vi "ELVIS III v1.0 Get Reset Actions.vi"(8 "error in":errorcluster, 11 "String":string) -> (0 "error out":errorcluster, 3 "Resources":string[](array[string]))   [LabVIEW 2021]
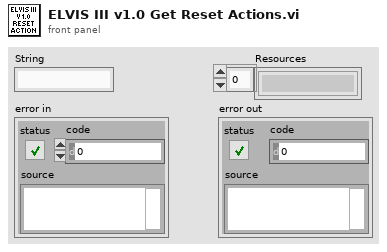
[diagram p1: front panel]
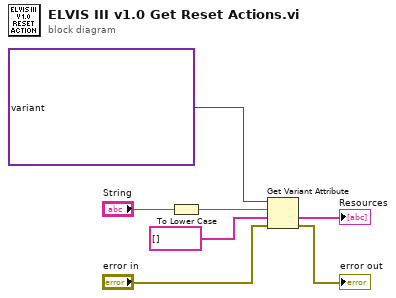
[diagram p0: block diagram]
diagram:
  n1 = To Lower Case(string="String") -> (all lower case string=w6:string)
  n2 = Get Variant Attribute(Variant=variant("a/ai0 (continuous)"=variant(string[] ["No"]), "a/ai0 (diff continuous)"=variant(string[] ["No"]), "a/ai0 (diff n samples)"=variant(string[] ["No"]), "a/ai0 (diff)"=variant(string[] ["No"]), "a/ai0 (interrupt)"=variant(string[] ["No"]), "a/ai0 (n samples)"=variant(string[] ["No"]), "a/ai1"=variant(string[] ["No"]), "a/ai1 (continuous)"=variant(string[] ["No"]), "a/ai1 (diff continuous)"=variant(string[] ["No"]), "a/ai1 (diff n samples)"=variant(string[] ["No"]), "a/ai1 (diff)"=variant(string[] ["No"]), "a/ai1 (interrupt)"=variant(string[] ["No"]), "a/ai1 (n samples)"=variant(string[] ["No"]), "a/ai2"=variant(string[] ["No"]), "a/ai2 (continuous)"=variant(string[] ["No"]), "a/ai2 (diff continuous)"=variant(string[] ["No"]), "a/ai2 (diff n samples)"=variant(string[] ["No"]), "a/ai2 (diff)"=variant(string[] ["No"]), "a/ai2 (n samples)"=variant(string[] ["No"]), "a/ai3"=variant(string[] ["No"]), "a/ai3 (continuous)"=variant(string[] ["No"]), "a/ai3 (diff continuous)"=variant(string[] ["No"]), "a/ai3 (diff n samples)"=variant(string[] ["No"]), "a/ai3 (diff)"=variant(string[] ["No"]), "a/ai3 (n samples)"=variant(string[] ["No"]), "a/ai4"=variant(string[] ["No"]), "a/ai4 (continuous)"=variant(string[] ["No"]), "a/ai4 (n samples)"=variant(string[] ["No"]), "a/ai5"=variant(string[] ["No"]), "a/ai5 (continuous)"=variant(string[] ["No"]), "a/ai5 (n samples)"=variant(string[] ["No"]), "a/ai6"=variant(string[] ["No"]), "a/ai6 (continuous)"=variant(string[] ["No"]), "a/ai6 (n samples)"=variant(string[] ["No"]), "a/ai7"=variant(string[] ["No"]), "a/ai7 (continuous)"=variant(string[] ["No"]), "a/ai7 (n samples)"=variant(string[] ["No"]), "a/ao0"=variant(string[] ["AO"]), "a/ao0 (continuous)"=variant(string[] ["AO DMA", "AO"]), "a/ao0 (n samples)"=variant(string[] ["AO"]), "a/ao1"=variant(string[] ["AO"]), "a/ao1 (continuous)"=variant(string[] ["AO DMA", "AO"]), "a/ao1 (n samples)"=variant(string[] ["AO"]), "a/di0 (n samples)"=variant(string[] ["DI N Samples"]), "a/di1 (n samples)"=variant(string[] ["DI N Samples"]), "a/di10 (n samples)"=variant(string[] ["DI N Samples"]), "a/di11 (n samples)"=variant(string[] ["DI N Samples"]), "a/di12 (n samples)"=variant(string[] ["DI N Samples"]), "a/di13 (n samples)"=variant(string[] ["DI N Samples"]), "a/di14 (n samples)"=variant(string[] ["DI N Samples"]), "a/di15 (n samples)"=variant(string[] ["DI N Samples"]), "a/di16 (n samples)"=variant(string[] ["DI N Samples"]), "a/di17 (n samples)"=variant(string[] ["DI N Samples"]), "a/di18 (n samples)"=variant(string[] ["DI N Samples"]), "a/di19 (n samples)"=variant(string[] ["DI N Samples"]), "a/di2 (n samples)"=variant(string[] ["DI N Samples"]), "a/di3 (n samples)"=variant(string[] ["DI N Samples"]), "a/di4 (n samples)"=variant(string[] ["DI N Samples"]), "a/di5 (n samples)"=variant(string[] ["DI N Samples"]), "a/di6 (n samples)"=variant(string[] ["DI N Samples"]), "a/di7 (n samples)"=variant(string[] ["DI N Samples"]), "a/di8 (n samples)"=variant(string[] ["DI N Samples"]), "a/di9 (n samples)"=variant(string[] ["DI N Samples"]), "a/dio0"=variant(string[] ["DIO"]), "a/dio0 (interrupt)"=variant(string[] ["No"]), "a/dio1"=variant(string[] ["DIO"]), "a/dio1 (interrupt)"=variant(string[] ["No"]), "a/dio10"=variant(string[] ["DIO"]), "a/dio11"=variant(string[] ["DIO"]), "a/dio12"=variant(string[] ["DIO"]), "a/dio13"=variant(string[] ["DIO"]), "a/dio14"=variant(string[] ["DIO"]), "a/dio15"=variant(string[] ["DIO"]), "a/dio16"=variant(string[] ["DIO"]), "a/dio17"=variant(string[] ["DIO"]), "a/dio18"=variant(string[] ["DIO"]), "a/dio19"=variant(string[] ["DIO"]), "a/dio2"=variant(string[] ["DIO"]), "a/dio2 (interrupt)"=variant(string[] ["No"]), "a/dio3"=variant(string[] ["DIO"]), "a/dio3 (interrupt)"=variant(string[] ["No"]), "a/dio4"=variant(string[] ["DIO"]), "a/dio5"=variant(string[] ["DIO"]), "a/dio6"=variant(string[] ["DIO"]), "a/dio7"=variant(string[] ["DIO"]), "a/dio8"=variant(string[] ["DIO"]), "a/dio9"=variant(string[] ["DIO"]), "a/do0 (n samples)"=variant(string[] ["DO N Samples"]), "a/do1 (n samples)"=variant(string[] ["DO N Samples"]), "a/do10 (n samples)"=variant(string[] ["DO N Samples"]), "a/do11 (n samples)"=variant(string[] ["DO N Samples"]), "a/do12 (n samples)"=variant(string[] ["DO N Samples"]), "a/do13 (n samples)"=variant(string[] ["DO N Samples"]), "a/do14 (n samples)"=variant(string[] ["DO N Samples"]), "a/do15 (n samples)"=variant(string[] ["DO N Samples"]), "a/do16 (n samples)"=variant(string[] ["DO N Samples"]), "a/do17 (n samples)"=variant(string[] ["DO N Samples"]), "a/do18 (n samples)"=variant(string[] ["DO N Samples"]), "a/do19 (n samples)"=variant(string[] ["DO N Samples"]), "a/do2 (n samples)"=variant(string[] ["DO N Samples"]), "a/do3 (n samples)"=variant(string[] ["DO N Samples"]), "a/do4 (n samples)"=variant(string[] ["DO N Samples"]), "a/do5 (n samples)"=variant(string[] ["DO N Samples"]), "a/do6 (n samples)"=variant(string[] ["DO N Samples"]), "a/do7 (n samples)"=variant(string[] ["DO N Samples"]), "a/do8 (n samples)"=variant(string[] ["DO N Samples"]), "a/do9 (n samples)"=variant(string[] ["DO N Samples"]), "a/enc0"=variant(string[] ["ENC"]), "a/enc1"=variant(string[] ["ENC"]), "a/enc2"=variant(string[] ["ENC"]), "a/enc3"=variant(string[] ["ENC"]), "a/enc4"=variant(string[] ["ENC"]), "a/enc5"=variant(string[] ["ENC"]), "a/enc6"=variant(string[] ["ENC"]), "a/enc7"=variant(string[] ["ENC"]), "a/enc8"=variant(string[] ["ENC"]), "a/enc9"=variant(string[] ["ENC"]), "a/i2c"=variant(string[] ["I2C"]), "a/pwm0"=variant(string[] ["PWM"]), "a/pwm1"=variant(string[] ["PWM"]), "a/pwm10"=variant(string[] ["PWM"]), "a/pwm11"=variant(string[] ["PWM"]), "a/pwm12"=variant(string[] ["PWM"]), "a/pwm13"=variant(string[] ["PWM"]), "a/pwm14"=variant(string[] ["PWM"]), "a/pwm15"=variant(string[] ["PWM"]), "a/pwm16"=variant(string[] ["PWM"]), "a/pwm17"=variant(string[] ["PWM"]), "a/pwm18"=variant(string[] ["PWM"]), "a/pwm19"=variant(string[] ["PWM"]), "a/pwm2"=variant(string[] ["PWM"]), "a/pwm3"=variant(string[] ["PWM"]), "a/pwm4"=variant(string[] ["PWM"]), "a/pwm5"=variant(string[] ["PWM"]), "a/pwm6"=variant(string[] ["PWM"]), "a/pwm7"=variant(string[] ["PWM"]), "a/pwm8"=variant(string[] ["PWM"]), "a/pwm9"=variant(string[] ["PWM"]), "a/spi"=variant(string[] ["SPI"]), "asrl1::instr"=variant(string[] ["UART"]), "asrl2::instr"=variant(string[] ["UART"]), "b/ai0"=variant(string[] ["No"]), "b/ai0 (continuous)"=variant(string[] ["No"]), "b/ai0 (diff continuous)"=variant(string[] ["No"]), "b/ai0 (diff n samples)"=variant(string[] ["No"]), "b/ai0 (diff)"=variant(string[] ["No"]), "b/ai0 (n samples)"=variant(string[] ["No"]), "b/ai1"=variant(string[] ["No"]), "b/ai1 (continuous)"=variant(string[] ["No"]), "b/ai1 (diff continuous)"=variant(string[] ["No"]), "b/ai1 (diff n samples)"=variant(string[] ["No"]), "b/ai1 (diff)"=variant(string[] ["No"]), "b/ai1 (n samples)"=variant(string[] ["No"]), "b/ai2"=variant(string[] ["No"]), "b/ai2 (continuous)"=variant(string[] ["No"]), "b/ai2 (diff continuous)"=variant(string[] ["No"]), "b/ai2 (diff n samples)"=variant(string[] ["No"]), "b/ai2 (diff)"=variant(string[] ["No"]), "b/ai2 (n samples)"=variant(string[] ["No"]), "b/ai3"=variant(string[] ["No"]), "b/ai3 (continuous)"=variant(string[] ["No"]), "b/ai3 (diff continuous)"=variant(string[] ["No"]), "b/ai3 (diff n samples)"=variant(string[] ["No"]), "b/ai3 (diff)"=variant(string[] ["No"]), "b/ai3 (n samples)"=variant(string[] ["No"]), "b/ai4"=variant(string[] ["No"]), "b/ai4 (continuous)"=variant(string[] ["No"]), "b/ai4 (n samples)"=variant(string[] ["No"]), "b/ai5"=variant(string[] ["No"]), "b/ai5 (continuous)"=variant(string[] ["No"]), "b/ai5 (n samples)"=variant(string[] ["No"]), "b/ai6"=variant(string[] ["No"]), "b/ai6 (continuous)"=variant(string[] ["No"]), "b/ai6 (n samples)"=variant(string[] ["No"]), "b/ai7"=variant(string[] ["No"]), "b/ai7 (continuous)"=variant(string[] ["No"]), "b/ai7 (n samples)"=variant(string[] ["No"]), "b/ao0"=variant(string[] ["AO"]), "b/ao0 (continuous)"=variant(string[] ["AO DMA", "AO"]), "b/ao0 (n samples)"=variant(string[] ["AO"]), "b/ao1"=variant(string[] ["AO"]), "b/ao1 (continuous)"=variant(string[] ["AO DMA", "AO"]), "b/ao1 (n samples)"=variant(string[] ["AO"]), "b/di0 (n samples)"=variant(string[] ["DI N Samples"]), "b/di1 (n samples)"=variant(string[] ["DI N Samples"]), "b/di10 (n samples)"=variant(string[] ["DI N Samples"]), "b/di11 (n samples)"=variant(string[] ["DI N Samples"]), "b/di12 (n samples)"=variant(string[] ["DI N Samples"]), "b/di13 (n samples)"=variant(string[] ["DI N Samples"]), "b/di14 (n samples)"=variant(string[] ["DI N Samples"]), "b/di15 (n samples)"=variant(string[] ["DI N Samples"]), "b/di16 (n samples)"=variant(string[] ["DI N Samples"]), "b/di17 (n samples)"=variant(string[] ["DI N Samples"]), "b/di18 (n samples)"=variant(string[] ["DI N Samples"]), "b/di19 (n samples)"=variant(string[] ["DI N Samples"]), "b/di2 (n samples)"=variant(string[] ["DI N Samples"]), "b/di3 (n samples)"=variant(string[] ["DI N Samples"]), "b/di4 (n samples)"=variant(string[] ["DI N Samples"]), "b/di5 (n samples)"=variant(string[] ["DI N Samples"]), "b/di6 (n samples)"=variant(string[] ["DI N Samples"]), "b/di7 (n samples)"=variant(string[] ["DI N Samples"]), "b/di8 (n samples)"=variant(string[] ["DI N Samples"]), "b/di9 (n samples)"=variant(string[] ["DI N Samples"]), "b/dio0"=variant(string[] ["DIO"]), "b/dio1"=variant(string[] ["DIO"]), "b/dio10"=variant(string[] ["DIO"]), "b/dio11"=variant(string[] ["DIO"]), "b/dio12"=variant(string[] ["DIO"]), "b/dio13"=variant(string[] ["DIO"]), "b/dio14"=variant(string[] ["DIO"]), "b/dio15"=variant(string[] ["DIO"]), "b/dio16"=variant(string[] ["DIO"]), "b/dio17"=variant(string[] ["DIO"]), "b/dio18"=variant(string[] ["DIO"]), "b/dio19"=variant(string[] ["DIO"]), "b/dio2"=variant(string[] ["DIO"]), "b/dio3"=variant(string[] ["DIO"]), "b/dio4"=variant(string[] ["DIO"]), "b/dio5"=variant(string[] ["DIO"]), "b/dio6"=variant(string[] ["DIO"]), "b/dio7"=variant(string[] ["DIO"]), "b/dio8"=variant(string[] ["DIO"]), "b/dio9"=variant(string[] ["DIO"]), "b/do0 (n samples)"=variant(string[] ["DO N Samples"]), "b/do1 (n samples)"=variant(string[] ["DO N Samples"]), "b/do10 (n samples)"=variant(string[] ["DO N Samples"]), "b/do11 (n samples)"=variant(string[] ["DO N Samples"]), "b/do12 (n samples)"=variant(string[] ["DO N Samples"]), "b/do13 (n samples)"=variant(string[] ["DO N Samples"]), "b/do14 (n samples)"=variant(string[] ["DO N Samples"]), "b/do15 (n samples)"=variant(string[] ["DO N Samples"]), "b/do16 (n samples)"=variant(string[] ["DO N Samples"]), "b/do17 (n samples)"=variant(string[] ["DO N Samples"]), "b/do18 (n samples)"=variant(string[] ["DO N Samples"]), "b/do19 (n samples)"=variant(string[] ["DO N Samples"]), "b/do2 (n samples)"=variant(string[] ["DO N Samples"]), "b/do3 (n samples)"=variant(string[] ["DO N Samples"]), "b/do4 (n samples)"=variant(string[] ["DO N Samples"]), "b/do5 (n samples)"=variant(string[] ["DO N Samples"]), "b/do6 (n samples)"=variant(string[] ["DO N Samples"]), "b/do7 (n samples)"=variant(string[] ["DO N Samples"]), "b/do8 (n samples)"=variant(string[] ["DO N Samples"]), "b/do9 (n samples)"=variant(string[] ["DO N Samples"]), "b/enc0"=variant(string[] ["ENC"]), "b/enc1"=variant(string[] ["ENC"]), "b/enc2"=variant(string[] ["ENC"]), "b/enc3"=variant(string[] ["ENC"]), "b/enc4"=variant(string[] ["ENC"]), "b/enc5"=variant(string[] ["ENC"]), "b/enc6"=variant(string[] ["ENC"]), "b/enc7"=variant(string[] ["ENC"]), "b/enc8"=variant(string[] ["ENC"]), "b/enc9"=variant(string[] ["ENC"]), "b/i2c"=variant(string[] ["I2C"]), "b/pwm0"=variant(string[] ["PWM"]), "b/pwm1"=variant(string[] ["PWM"]), "b/pwm10"=variant(string[] ["PWM"]), "b/pwm11"=variant(string[] ["PWM"]), "b/pwm12"=variant(string[] ["PWM"]), "b/pwm13"=variant(string[] ["PWM"]), "b/pwm14"=variant(string[] ["PWM"]), "b/pwm15"=variant(string[] ["PWM"]), "b/pwm16"=variant(string[] ["PWM"]), "b/pwm17"=variant(string[] ["PWM"]), "b/pwm18"=variant(string[] ["PWM"]), "b/pwm19"=variant(string[] ["PWM"]), "b/pwm2"=variant(string[] ["PWM"]), "b/pwm3"=variant(string[] ["PWM"]), "b/pwm4"=variant(string[] ["PWM"]), "b/pwm5"=variant(string[] ["PWM"]), "b/pwm6"=variant(string[] ["PWM"]), "b/pwm7"=variant(string[] ["PWM"]), "b/pwm8"=variant(string[] ["PWM"]), "b/pwm9"=variant(string[] ["PWM"]), "b/spi"=variant(string[] ["SPI"]), "button0"=variant(string[] ["DIO"]), "button0 (interrupt)"=variant(string[] ["No"]), "led0"=variant(string[] ["DIO"]), "led1"=variant(string[] ["DIO"]), "led2"=variant(string[] ["DIO"]), "led3"=variant(string[] ["DIO"]), "﻿a/ai0"=variant(string[] ["No"])) ("RIO Resource Map"), name=w6, default value (empty Variant)=string[] [] ("Resources"), error in="error in") -> (value=→"Resources":string[], error out=→"error out":errorcluster)  [unwired: 2 out]
